vi "CAN_SetControlMode.vi"(8 "error in (no error)":errorcluster, 10 "Control Mode":T3, 11 "CAN Jaguars Ref":T1) -> (0 "error out":errorcluster, 3 "CAN Jaguars Ref out":T1)   [LabVIEW 2009, in "OWNCAN.lvlib"]
doc: "Sets the control mode of Jaguars (Voltage, Current, Speed or Position)"
uses:
  OWNCAN.lvlib
  CAN/SubVIs/CAN Jaguar Control Mode.ctl
  CAN Jaguars Ref.ctl
  CAN/SubVIs/CAN Jaguar Ref.ctl
  CAN.lvlib
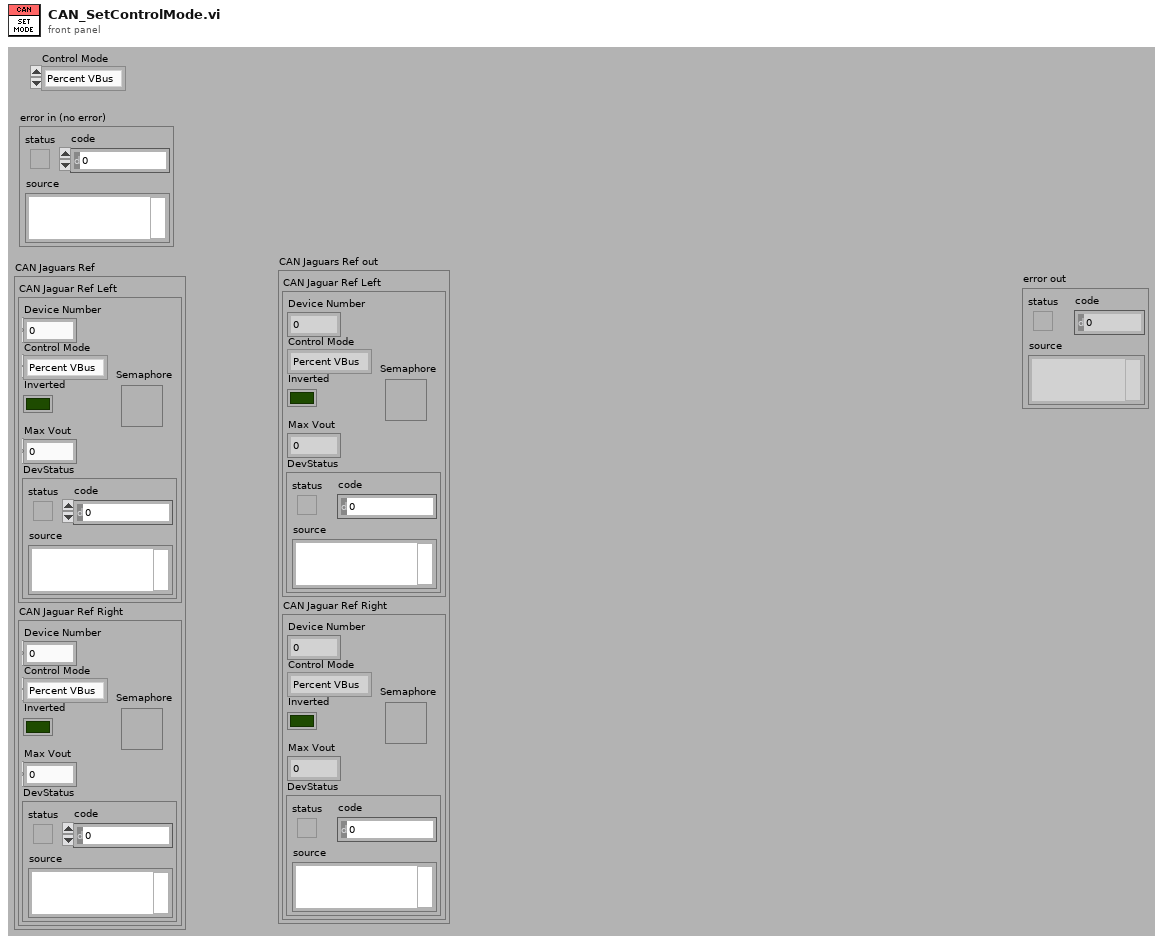
[diagram p1: front panel]
types:
  T1 = typedef "OWNCAN.lvlib/CAN Jaguars Ref.ctl" = cluster{"CAN Jaguar Ref Left":T2, "CAN Jaguar Ref Right":T2}
  T2 = typedef "CAN.lvlib/CAN Jaguar Ref.ctl" = cluster{"Device Number":u8, "Control Mode":T3, "Inverted":bool, "Semaphore":T4, "Max Vout":dbl, "DevStatus":errorcluster}
  T3 = typedef "CAN.lvlib/CAN Jaguar Control Mode.ctl" = enum16{"Percent VBus", "Speed", "Position", "Current"}
  T4 = typedef "Semaphore RefNum" = refnum<k1>
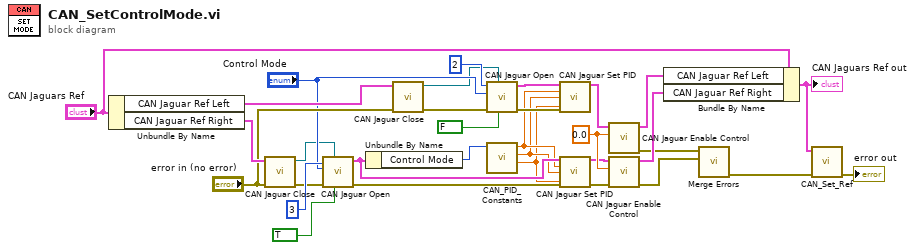
[diagram p0: block diagram]
diagram:
  w28 = 0.0 ("Encoder Initial Position")
  n1 = Unbundle By Name("CAN Jaguars Ref") -> ("CAN Jaguar Ref Left"=w27:T2, "CAN Jaguar Ref Right"=w26:T2)
  n2 = call "CAN Jaguar Close.vi"("error in (no error)"="error in (no error)", "CAN Jaguar Ref"=w26) -> ("error out"=w23:errorcluster, "Semaphore"=w4:T4)  [unwired: 8 in]
  n3 = call "CAN Jaguar Open.vi"("Inverted"=TRUE, "Semaphore"=w4, "error in (no error)"=w23, "Control Mode"="Control Mode", "Device Number"=u8 3) -> ("error out"=w12:errorcluster, "CAN Jaguar Ref Out"=w13:T2)  [unwired: 5 in]
  n4 = Unbundle By Name(w13) -> ("Control Mode"=w17:T3)
  n5 = call "CAN Jaguar Close.vi"("error in (no error)"="error in (no error)", "CAN Jaguar Ref"=w27) -> ("error out"=w24:errorcluster, "Semaphore"=w5:T4)  [unwired: 8 in]
  n6 = call "CAN Jaguar Open.vi"("Inverted"=FALSE, "Semaphore"=w5, "error in (no error)"=w24, "Control Mode"="Control Mode", "Device Number"=u8 2) -> ("error out"=w10:errorcluster, "CAN Jaguar Ref Out"=w16:T2)  [unwired: 5 in]
  n7 = call "CAN_PID_Constants.vi"("Control Mode"=w17) -> ("D"=w7:dbl, "I"=w8:dbl, "P"=w9:dbl)  [unwired: 8 in]
  n8 = call "CAN Jaguar Set PID.vi"("CAN Jaguar Ref"=w16, "P"=w9, "I"=w8, "D"=w7, "error in (no error)"=w10) -> ("CAN Jaguar Ref Out"=w15:T2)  [unwired: 9 in, 1 out]
  n9 = call "CAN Jaguar Set PID.vi"("CAN Jaguar Ref"=w13, "P"=w9, "I"=w8, "D"=w7, "error in (no error)"=w12) -> ("CAN Jaguar Ref Out"=w14:T2, "error out"=w11:errorcluster)  [unwired: 9 in]
  n10 = call "CAN Jaguar Enable Control.vi"("Encoder Initial Position"=w28, "CAN Jaguar Ref"=w15) -> ("error out"=w19:errorcluster, "CAN Jaguar Ref Out"=w21:T2)  [unwired: 8 in]
  n11 = call "CAN Jaguar Enable Control.vi"("error in (no error)"=w11, "Encoder Initial Position"=w28, "CAN Jaguar Ref"=w14) -> ("error out"=w18:errorcluster, "CAN Jaguar Ref Out"=w20:T2)  [unwired: 7 in]
  n12 = Bundle By Name(cluster="CAN Jaguars Ref", "CAN Jaguar Ref Left"=w21, "CAN Jaguar Ref Right"=w20) -> (w3:T1)
  "CAN Jaguars Ref out" <- w3
  n13 = call <vilib>:"Merge Errors.vi"("error in 2 (no error)"=w18, "error in 1 (no error)"=w19) -> ("error out"=w2:errorcluster)  [unwired: 5 in]
  n14 = call "CAN_Set_Ref.vi"("error in (no error)"=w2, "CAN_Jaguars_ref"=w3) -> ("error out"=→"error out":errorcluster)  [unwired: 9 in]
